vi "HFRR ADV v024 new software.vi"() -> ()   [LabVIEW 2025] (continued)
            n3097 = local write "OK Button 17"(FALSE ("OK Button 17")) -> ()
            n3098 = local read "String"() -> (w4300:string)
            n3099 = String To Path(string=w4300) -> (path=w4301:path)
            n3100 = File Dialog(6:"*.duf" ("pattern"), 7:w4305, 11:w4301) -> (0:w4292:errorcluster, 3:w4311:path)  [unwired: 4 in, 2 out]
            n3101 = Unbundle(w4292) -> ()  [unwired: 3 out]
            n3102 = Open/Create/Replace File "Open File"(file path (use dialog)=w4311) -> (refnum out=w4303:refnum<file>)  [unwired: 5 in, 2 out]
            n3103 = Strip Path(path=w4311) -> (name=w4309:string)  [unwired: 1 out]
            n3104 = Path To String(path=w4311) -> (string=w4294:string)
            n3105 = while {
              tunnel: w4303 -> [w4315]
              i -> [w4312]
              stop <- w4313 continue-if-true
              (unwired) TRUE ("line mode (F)")
              n3106 = Read from Text File "Read File"(file (use dialog)=w4315) -> (text=w4314:string)  [unwired: 3 in, 3 out]
              n3107 = local write "Numeric 16"(w4312) -> ()
              n3108 = String Length(string=w4314) -> (length=w4317:i32)
              n3109 = Greater?(x=w4317, y=1) -> (0:w4313:bool)
            }
            n3110 = local write "String 29"(w4294) -> ()
            n3111 = Search and Replace String(input string=w4294, search string=".duf", replace string=".dgf" ("replace string (\"\")")) -> (result string=→"String Indicator 4":string)  [unwired: 5 in, 3 out]
            n3112 = Match Pattern(string=w4309, regular expression=".dwm") -> (before substring=w4293:string)  [unwired: 1 in, 3 out]
            "String Indicator" <- w4293
            n3113 = Match Pattern(string=w4294, regular expression=".dwm" ("substring (\"\")")) -> (before substring=w4295:string)  [unwired: 1 in, 3 out]
            "String Indicator 3" <- w4295
            n3114 = local write "TITTLE 2"(w4293) -> ()
            n3115 = String To Path(string=w4295) -> (path=w4302:path)
            "path" <- w4302
            n3116 = call <vilib>:"Read Characters From File.vi"("file path (dialog if empty)"=w4302, "start of read offset (chars.:0)"=60 ("start of read offset (chars.: 0)")) -> ("character string"=→"String Indicator 2":string)  [unwired: 4 in, 3 out]
          }
        }
        n3117 = call <vilib>:"Query Available Printers.vi"() -> ("system configured printers"=w3994:string[])  [unwired: 9 in, 2 out]
        "System Configured Printers 2" <- w3994
        n3118 = local read "OK Button 16"() -> (w3991:bool)
        n3119 = case shown="True" "OK Button 16" {
          frame False {
          }
          frame True {
            n3120 = stacked-sequence {
              frame #0 {
                n3121 = local read "Numeric 16"() -> (w4319:i32)
                n3122 = local write "Numeric 10"(w4319) -> ()
              }
              frame #1 {
                n3123 = local read "S.NO"() -> (→"s.NO":string)
                n3124 = local read "String 29"() -> (w4323:string)
                n3125 = String To Path(string=w4323) -> (path=w4322:path)
                n3126 = Open/Create/Replace File "Open File"(file path (use dialog)=w4322) -> (refnum out=w4324:refnum<file>)  [unwired: 5 in, 2 out]
                n3127 = for {
                  N: 16 -> [_]
                  tunnel: w4324 -> [w4331]
                  i -> [w4327]
                  (unwired) TRUE ("line mode (F)")
                  n3128 = Read from Text File "Read File"(file (use dialog)=w4331) -> (text=w4325:string)  [unwired: 3 in, 3 out]
                  n3129 = Match Pattern(string=w4325, regular expression="(") -> (after substring=w4330:string)  [unwired: 1 in, 3 out]
                  n3130 = Match Pattern(string=w4330, regular expression=")") -> (before substring=w4326:string)  [unwired: 1 in, 3 out]
                  n3131 = case shown="1" w4327 {
                    tunnel: w4326 -> [w4332 w4333 _ _ w4334 w4335 w4336 w4338 w4340 w4342 w4344 w4346 w4348 w4350 _]
                    tunnel: w4325 -> [_ _ _ _ _ _ _ _ _ _ _ _ _ _ _]
                    frame 0 {
                      "TITTLE" <- w4332
                    }
                    frame 1 {
                      "Sample ID" <- w4333
                    }
                    frame 2 {
                    }
                    frame 3 {
                    }
                    frame 4 {
                      "Test Date" <- w4334
                    }
                    frame 5 {
                      "Tested by" <- w4335
                    }
                    frame 6 {
                      n3132 = Fract/Exp String To Number(string=w4336) -> (number=→"Humidity before test 2":dbl)  [unwired: 3 in, 1 out]
                    }
                    frame 7 {
                      n3133 = Fract/Exp String To Number(string=w4338) -> (number=→"Temperature before test 2":dbl)  [unwired: 3 in, 1 out]
                    }
                    frame 8 {
                      n3134 = Fract/Exp String To Number(string=w4340) -> (number=→"Humidity after test 2":dbl)  [unwired: 3 in, 1 out]
                    }
                    frame 9 {
                      n3135 = Fract/Exp String To Number(string=w4342) -> (number=→"Temperature after test 2":dbl)  [unwired: 3 in, 1 out]
                    }
                    frame 10 {
                      n3136 = Fract/Exp String To Number(string=w4344) -> (number=→"MWSD 2":dbl)  [unwired: 3 in, 1 out]
                    }
                    frame 11 {
                      n3137 = Fract/Exp String To Number(string=w4346) -> (number=→"AVP 2":dbl)  [unwired: 3 in, 1 out]
                    }
                    frame 12 {
                      n3138 = Fract/Exp String To Number(string=w4348) -> (number=→"HCF 2":dbl)  [unwired: 3 in, 1 out]
                    }
                    frame 13 {
                      n3139 = Fract/Exp String To Number(string=w4350) -> (number=→"WS1.4 2":dbl)  [unwired: 3 in, 1 out]
                    }
                    frame 14, Default {
                    }
                  }
                }
              }
              frame #2 {
              }
            }
            n3140 = local write "OK Button 16"(FALSE ("OK Button 13")) -> ()
          }
        }
        n3141 = Index Array(array=w3994, index="Select Printer 3") -> (element=w3996:string)
        "Selected Printer" <- w3996
        n3142 = case shown="True" w3991 {
          frame False {
          }
          frame True {
            n3143 = flat-sequence {
              frame #0 {
              }
              frame #1 {
                n3144 = Wait (ms)(milliseconds to wait=u32 100) -> ()  [unwired: 1 out]
              }
              frame #2 {
                n3145 = local write "OK Button 16"(FALSE ("Print 3")) -> ()
              }
            }
          }
        }
        n3146 = case shown="True" "Print" {
          tunnel: w3996 -> [_ w4288]
          frame False {
          }
          frame True {
            (unwired) i16 6 ("width (-)")
            (unwired) "TESTED BY : "
            (unwired) "TESTED DATE :"
            (unwired) "SAMPLE ID : "
            (unwired) "SAMPLE DESIGN : "
            w4246 = "\r"
            w4263 = "\r"
            # "add image"
            n3147 = local read "Sample ID"() -> (w4236:string)
            n3148 = local read "Tested by"() -> (w4239:string)
            n3149 = local read "String 34"() -> (w4226:string)
            n3150 = local read "String 45"() -> (w4206:string)
            n3151 = local read "String 35"() -> (w4221:string)
            n3152 = local read "String 37"() -> (w4219:string)
            n3153 = local read "String 32"() -> (w4241:string)
            n3154 = local read "String 36"() -> (w4216:string)
            n3155 = local read "String 31"() -> (w4240:string)
            n3156 = local read "Test Date"() -> (w4237:string)
            n3157 = local read "String 33"() -> (w4242:string)
            n3158 = local read "String 38"() -> (w4212:string)
            n3159 = local read "String 39"() -> (w4209:string)
            n3160 = local write "Print"(FALSE ("Print FF")) -> ()
            n3161 = local read "S 39"() -> (w4224:string)
            n3162 = local read "S 38"() -> (w4231:string)
            n3163 = local read "Temperature before test 2"() -> (w4262:dbl)
            n3164 = local read "Temperature after test 2"() -> (w4252:dbl)
            n3165 = local read "Humidity before test 2"() -> (w4277:dbl)
            n3166 = local read "Humidity after test 2"() -> (w4261:dbl)
            n3167 = local read "MWSD 2"() -> (w4266:dbl)
            n3168 = local read "WS1.4 2"() -> (w4244:dbl)
            n3169 = Concatenate Strings("2)" ("string"), w4226) -> (w4227:string)
            n3170 = Concatenate Strings("3)" ("string"), w4224) -> (w4225:string)
            n3171 = Concatenate Strings("1)" ("string"), w4231) -> (w4230:string)
            n3172 = Concatenate Strings("4)" ("string"), w4221) -> (w4222:string)
            n3173 = Concatenate Strings("5)" ("string"), w4219) -> (w4218:string)
            n3174 = Concatenate Strings("6)" ("string"), w4216) -> (w4215:string)
            n3175 = Concatenate Strings("7)" ("string"), w4212) -> (w4213:string)
            n3176 = Concatenate Strings("8)" ("string"), w4209) -> (w4210:string)
            n3177 = local read "HCF 2"() -> (w4248:dbl)
            n3178 = local read "AVP 2"() -> (w4265:dbl)
            n3179 = local read "s.NO"() -> (w4207:string)
            n3180 = call <vilib>:"New Report.vi"("report type"=enum16{"Standard Report", "HTML"}."Standard Report") -> ("report out"=w4286:refnum<class "NI_report.lvclass">, "error out"=w4285:errorcluster)  [unwired: 13 in]
            n3181 = local read "TITTLE"() -> (w4238:string)
            n3182 = Concatenate Strings(w4263, w4206, w4207, w4263, w4241, w4236, w4263, w4240, w4237, w4263, w4242, w4239, w4263) -> (w4256:string)
            "test by" <- w4256
            n3183 = Number To Fractional String(number=w4262, width (-)=i16 6, precision (6)=i16 2) -> (F-format string=w4251:string)  [unwired: 1 in]
            n3184 = Number To Fractional String(number=w4261, width (-)=i16 6, precision (6)=i16 2) -> (F-format string=w4264:string)  [unwired: 1 in]
            n3185 = Number To Fractional String(number=w4277, width (-)=i16 6, precision (6)=i16 2) -> (F-format string=w4282:string)  [unwired: 1 in]
            n3186 = Number To Fractional String(number=w4266, width (-)=i16 6, precision (6)=i16 2) -> (F-format string=w4268:string)  [unwired: 1 in]
            n3187 = Number To Fractional String(number=w4252, width (-)=i16 6, precision (6)=i16 2) -> (F-format string=w4253:string)  [unwired: 1 in]
            n3188 = Number To Fractional String(number=w4265, width (-)=i16 6, precision (6)=i16 2) -> (F-format string=w4267:string)  [unwired: 1 in]
            n3189 = Number To Fractional String(number=w4248, width (-)=i16 6, precision (6)=i16 2) -> (F-format string=w4247:string)  [unwired: 1 in]
            n3190 = Number To Fractional String(number=w4244, precision (6)=i16 2) -> (F-format string=w4243:string)  [unwired: 2 in]
            n3191 = call-dynamic "Set Report Header Text.vi"("report in"=w4286, "center header text"=w4238, "error in (no error)"=w4285) -> ("report out"=w4257:refnum<class "NI_report.lvclass">, "error out"=w4258:errorcluster)  [unwired: 11 in]
            n3192 = Concatenate Strings(w4246, w4230, w4282, w4246, w4227, w4251, w4246, w4225, w4264, w4246, w4222, w4253, w4246, w4218, w4268, w4246, w4215, w4267, w4246, w4213, w4247, w4246, w4210, w4243) -> (w4234:string)
            "export 2" <- w4234
            n3193 = call-poly <vilib>:"Append Report Text.vi"("report in"=w4257, "text"=w4256, "error in (no error)"=w4258) -> ("report out"=w4260:refnum<class "NI_report.lvclass">, "error out"=w4259:errorcluster)  [unwired: 9 in, 2 out]
            n3194 = local read "test by"() -> (w4233:string)
            n3195 = local read "TITTLE"() -> (w4235:string)
            n3196 = call-poly <vilib>:"Append Report Text.vi"("report in"=w4260, "error in (no error)"=w4259) -> ("report out"=w4281:refnum<class "NI_report.lvclass">, "error out"=w4279:errorcluster)  [unwired: 10 in, 2 out]
            n3197 = Concatenate Strings(w4235, w4234, w4233) -> (→"output":string)
            n3198 = call-poly <vilib>:"Append Report Text.vi"("report in"=w4281, "text"=w4234, "error in (no error)"=w4279) -> ("report out"=w4280:refnum<class "NI_report.lvclass">, "error out"=w4278:errorcluster)  [unwired: 9 in, 2 out]
            n3199 = call-dynamic "Print Report.vi"("report in"=w4280, "printer name (default)"=w4288, "error in (no error)"=w4278) -> ("report out"=w4290:refnum<class "NI_report.lvclass">, "error out"=w4291:errorcluster)  [unwired: 11 in]
            n3200 = call-dynamic "Dispose Report.vi"("report in"=w4290, "error in (no error)"=w4291) -> ()  [unwired: 13 in, 1 out]
          }
        }
        n3201 = case shown="True" "Print 2" {
          frame False {
          }
          frame True {
            n3202 = flat-sequence {
              frame #0 {
                n3203 = local read "s.NO"() -> (→"s.NO 2":string)
                n3204 = Wait (ms)(milliseconds to wait=u32 20) -> ()  [unwired: 1 out]
                n3205 = local read "Sample ID  3"() -> (→"Sample ID  6":string)
                n3206 = local read "Sample ID  4"() -> (→"Sample ID  7":string)
                n3207 = local read "Sample ID"() -> (→"Sample ID  2":string)
                n3208 = local read "Tested by"() -> (→"Tested by 2":string)
                n3209 = local read "Test Date"() -> (→"Test Date 2":string)
                n3210 = local read "Humidity after test 3"() -> (→"Humidity after test 4":dbl)
                n3211 = local read "Ref A Test Date :"() -> (→"TITTLE 4":string)
                n3212 = local read "Temperature before test 3"() -> (w4113:dbl)
                n3213 = local read "Temperature before test 3"() -> (→"Temperature after test 5":dbl)
                n3214 = local read "Temperature after test 3"() -> (→"Temperature after test 4":dbl)
                n3215 = local read "Humidity before test 3"() -> (→"Humidity before test 4":dbl)
                n3216 = local write "Temperature before test 3"(w4113) -> ()
                n3217 = local read "image data"() -> (w4104:T16)
                n3218 = String To Path(string="C:\\LAB-IQ\\im\\Temp_resized.jpg") -> (path=w4105:path)
                "path 2" <- w4105
                n3219 = call <vilib>:"Write JPEG File.vi"("image data"=w4104, "path to JPEG file"=w4105) -> ()  [unwired: 8 in, 2 out]
                "Ref A Test Date :" <- "Ref A Test Date :"
                "Ref B Test Date :" <- "Ref B Test Date :"
                "Ref B Scar Value :" <- "Ref B Scar Value :"
                "Ref A Scar Value :" <- "Ref A Scar Value :"
              }
              frame #1 {
                (unwired) HTML_Report_Image_Alignment."MIDDLE" ("alignment (default)")
                w4141 = u16 0 items=["portrait", "landscape"] ("orientation (portrait)")
                (unwired) HTML_Report_Image_Alignment."ABSMIDDLE" ("alignment (default)")
                (unwired) "TESTED BY : "
                (unwired) "TESTED DATE :"
                (unwired) "SAMPLE ID : "
                (unwired) "SAMPLE DESIGN : "
                w4174 = "\r"
                # "add image"
                n3220 = Wait (ms)(milliseconds to wait=u32 20) -> ()  [unwired: 1 out]
                n3221 = local read "Sample ID  2"() -> (w4167:string)
                n3222 = local read "Wear Scar X"() -> (w4139:dbl)
                "Length ( microns ) 2" <- w4139
                n3223 = local read "Wear Scar Y"() -> (w4138:dbl)
                "Wear Scar Y ( microns ) :" <- w4138
                n3224 = local read "Test Date 2"() -> (w4168:string)
                n3225 = local read "Tested by 2"() -> (w4169:string)
                n3226 = local read "String 46"() -> (w4165:string)
                n3227 = local read "String 48"() -> (w4171:string)
                n3228 = local read "String 47"() -> (w4170:string)
                n3229 = local read "String 49"() -> (w4172:string)
                n3230 = local read "String 10"() -> (w4125:string)
                n3231 = local read "s.NO 2"() -> (w4166:string)
                n3232 = Add(x=w4139, y=w4138) -> (x+y=w4137:dbl)
                n3233 = call <vilib>:"New Report.vi"("report type"=enum16{"Standard Report", "HTML"}."HTML") -> ("report out"=w4145:refnum<class "NI_report.lvclass">, "error out"=w4143:errorcluster)  [unwired: 13 in]
                n3234 = Concatenate Strings(w4174, w4165, w4166, w4174, w4171, w4167, w4174, w4170, w4168, w4174, w4172, w4169, w4174) -> (→"test by 2":string)
                n3235 = Concatenate Strings("C:\\LAB-IQ\\Data\\" ("string"), w4125, ".jpg" ("string")) -> ()  [unwired: 1 out]
                n3236 = Divide(x=w4137, y=2.0) -> (x/y=→"Mean Wear ( microns) :":dbl)
                n3237 = call-dynamic "Set Report Orientation.vi"("report in"=w4145, "orientation (portrait)"=w4141, "error in (no error)"=w4143) -> ("report out"=w4144:refnum<class "NI_report.lvclass">, "error out"=w4142:errorcluster)  [unwired: 11 in]
                n3238 = for {
                  N: 5 -> [_]
                  tunnel: w4144 -> [w4195]
                  tunnel: [w4194] -> w4123
                  tunnel: w4142 -> [w4193]
                  tunnel: [w4192] -> w4122
                  n3239 = call-dynamic "Set Report Tab Width.vi"("report in"=w4195, "error in (no error)"=w4193) -> ("report out"=w4194:refnum<class "NI_report.lvclass">, "error out"=w4192:errorcluster)  [unwired: 12 in]
                }
                n3240 = local read "TITTLE"() -> (w4140:string)
                n3241 = call-dynamic "Set Report Header Text.vi"("report in"=w4123, "center header text"=w4140, "error in (no error)"=w4122) -> ("report out"=w4161:refnum<class "NI_report.lvclass">, "error out"=w4160:errorcluster)  [unwired: 11 in]
                n3242 = for {
                  N: 1 -> [_]
                  tunnel: [w4199] -> w4147
                  tunnel: [w4198] -> w4146
                  tunnel: w4161 -> [w4197]
                  tunnel: w4160 -> [w4196]
                  n3243 = call-dynamic "New Report Line.vi"("report in"=w4197, "error in (no error)"=w4196) -> ("report out"=w4199:refnum<class "NI_report.lvclass">, "error out"=w4198:errorcluster)  [unwired: 12 in]
                }
                n3244 = for {
                  N: 2 -> [_]
                  tunnel: [w4191] -> w4153
                  tunnel: [w4190] -> w4152
                  tunnel: w4147 -> [w4189]
                  tunnel: w4146 -> [w4188]
                  n3245 = call-dynamic "New Report Line.vi"("report in"=w4189, "error in (no error)"=w4188) -> ("report out"=w4191:refnum<class "NI_report.lvclass">, "error out"=w4190:errorcluster)  [unwired: 12 in]
                }
                n3246 = for {
                  N: 25 -> [_]
                  tunnel: w4153 -> [w4187]
                  tunnel: w4152 -> [w4185]
                  tunnel: [w4186] -> w4156
                  tunnel: [w4184] -> w4155
                  n3247 = call-dynamic "Set Report Tab Width.vi"("report in"=w4187, "error in (no error)"=w4185) -> ("report out"=w4186:refnum<class "NI_report.lvclass">, "error out"=w4184:errorcluster)  [unwired: 12 in]
                }
                n3248 = control-ref of="Tab Control 9"() -> (w4151:refnum<vi>)
                n3249 = call-dynamic "Append Control Image to Report.vi"("report in"=w4156, "alignment (default)"=HTML_Report_Image_Alignment."ABSMIDDLE", "ctrl reference"=w4151, "error in (no error)"=w4155) -> ("report out"=w4150:refnum<class "NI_report.lvclass">, "error out"=w4149:errorcluster)  [unwired: 8 in, 2 out]
                n3250 = for {
                  N: 3 -> [_]
                  tunnel: [w4183] -> w4134
                  tunnel: [w4182] -> w4133
                  tunnel: w4150 -> [w4181]
                  tunnel: w4149 -> [w4180]
                  n3251 = call-dynamic "New Report Line.vi"("report in"=w4181, "error in (no error)"=w4180) -> ("report out"=w4183:refnum<class "NI_report.lvclass">, "error out"=w4182:errorcluster)  [unwired: 12 in]
                }
                n3252 = for {
                  N: 100 -> [_]
                  tunnel: w4134 -> [w4179]
                  tunnel: w4133 -> [w4177]
                  tunnel: [w4178] -> w4130
                  tunnel: [w4176] -> w4128
                  n3253 = call-dynamic "Set Report Tab Width.vi"("report in"=w4179, "error in (no error)"=w4177) -> ("report out"=w4178:refnum<class "NI_report.lvclass">, "error out"=w4176:errorcluster)  [unwired: 12 in]
                }
                n3254 = String To Path(string="C:\\LAB-IQ\\im\\Temp_resized.jpg") -> (path=w4120:path)
                n3255 = call-poly <vilib>:"Append Image to Report.vi"("report in"=w4130, "path or URL of image"=w4120, "error in (no error)"=w4128) -> ("report out"=w4129:refnum<class "NI_report.lvclass">, "error out"=w4127:errorcluster)  [unwired: 9 in, 2 out]
                n3256 = call-poly <vilib>:"Open HTML Report in Browser.vi"("report in"=w4129, "error in (no error)"=w4127) -> ("report out"=w4164:refnum<class "NI_report.lvclass">, "error out"=w4163:errorcluster)  [unwired: 11 in, 1 out]
                n3257 = call-dynamic "Dispose Report.vi"("report in"=w4164, "error in (no error)"=w4163) -> ()  [unwired: 13 in, 1 out]
              }
              frame #2 {
              }
              frame #3 {
                n3258 = disable-structure shown="Disabled" {
                  frame Disabled {
                    n3259 = local read "String 10"() -> (w4204:string)
                    n3260 = Concatenate Strings("C:\\LAB-IQ-NXT\\Data\\" ("string"), w4204, ".jpg" ("string")) -> (w4202:string)
                    n3261 = String To Path(string=w4202) -> (path=w4201:path)
                    n3262 = Delete(path (use dialog)=w4201) -> ()  [unwired: 4 in, 3 out]
                  }
                  frame Enabled {
                  }
                }
                n3263 = local write "Print 2"(FALSE ("Print")) -> ()
              }
            }
          }
        }
      }
    }
    n3264 = property on="SetTemp" class="DigNum (strict)"("Disabled"=w2147) -> ()  [unwired: 2 in, 2 out]
    n3265 = Multiply(x=w2137, y=w2139) -> (x*y=w2138:dbl)
    n3266 = local read "MWSD"() -> (w2136:dbl)
    n3267 = Add(x=w2138, y=w2136) -> (x+y=→"WS1.4":dbl)
    n3268 = Wait (ms)(milliseconds to wait=u32 50) -> ()  [unwired: 1 out]
    n3269 = Wait (ms)(milliseconds to wait=u32 50) -> ()  [unwired: 1 out]
    n3270 = local read "Quit"() -> (w2135:bool)
  }
  n3271 = VISA Close(VISA resource name=w44, error in (no error)=w43) -> ()  [unwired: 1 out]
  n3272 = while {
    tunnel: [w4365] -> w53
    shift-right: [w4358] -> _
    shift-left: 0.0 -> [w4361]
    shift-right: [w4357] -> _
    shift-left: 0.0 -> [w4360]
    shift-right: [w4356] -> _
    shift-left: 100.0 ("vc_cmd") -> [w4359]
    stop <- w4365 stop-if-true
    # "PID LOGIC"
    n3273 = local read "RUN"() -> (w4363:bool)
    n3274 = local read "Auto Start Temp"() -> (w4352:bool)
    n3275 = local read "Auto Start Test"() -> (w4362:bool)
    n3276 = local read "START TEMP"() -> (w4354:bool)
    n3277 = And(x=w4352, y=w4362) -> (x .and. y?=w4353:bool)
    n3278 = Or(x=w4363, y=w4353) -> (x .or. y?=w4364:bool)
    n3279 = And(x=w4364, y=w4354) -> (x .and. y?=w4355:bool)
    n3280 = Wait (ms)(milliseconds to wait="milliseconds to wait") -> ()  [unwired: 1 out]
    n3281 = case shown="True" w4355 {
      tunnel: [400.0 ("out_vc_cmd") w4385] -> w4356
      tunnel: [w4368 w4387] -> w4357
      tunnel: [w4368 w4386] -> w4358
      tunnel: w4361 -> [_ w4376]
      tunnel: w4360 -> [_ w4375]
      tunnel: w4359 -> [_ w4374]
      frame False {
        w4368 = 0.0 ("error_out")
      }
      frame True {
        n3282 = local read "Set Strk"() -> (w4371:dbl)
        n3283 = local read "LVDT STROKE"() -> (w4369:dbl)
        n3284 = Add(x=w4371, y="Add up Stroke") -> (x+y=w4372:dbl)
        n3285 = formula code="// Zero-Hardcode Explicit Positional-Form PID Engine\n// Inputs: target_stroke, measured_stroke, dt, prev_error, integral_accumulator_in, prev_vc_cmd\n//         kp, ki, kd, max_step_change, max_amplitude, min_amplitude, startup_cmd\n// Outputs: vc_cmd, error_out, out_error, integral_accumulator_out, out_vc_cmd\n\n// 1. Calculate Tracking Error\nfloat current_error = target_stroke - measured_stroke;\nerror_out = current_error;\n\n// 2. Compute Proportional Term\nfloat p_term = kp * current_error;\n\n// 3. Compute Derivative Term\nfloat d_term = 0.0;\nif (dt > 0.0) {\n    d_term = kd * ((current_error - prev_error) / dt);\n}\n\n// 4. Update and Accumulate Integral Term\nfloat current_integral = integral_accumulator_in + (current_error * dt);\nfloat i_term = ki * current_integral;\n\n// 5. Calculate Ideal Target Command\nfloat ideal_command = startup_cmd + p_term + i_term + d_term;\n\n// 6. Anti-Windup Protection (Back-calculation method)\nif (ideal_command > max_amplitude) {\n    float excess = ideal_command - max_amplitude;\n    if (ki > 0.0) {\n        current_integral -= excess / ki;\n    }\n    ideal_command = max_amplitude;\n} else if (ideal_command < min_amplitude) {\n    float excess = ideal_command - min_amplitude;\n    if (ki > 0.0) {\n        current_integral -= excess / ki;\n    }\n    ideal_command = min_amplitude;\n}\n\n// 7. Apply Loop Rate Limiting (Protects voice coil from large voltage steps)\nfloat raw_adjustment = ideal_command - prev_vc_cmd;\n\nif (raw_adjustment > max_step_change) {\n    raw_adjustment = max_step_change;\n} else if (raw_adjustment < -max_step_change) {\n    raw_adjustment = -max_step_change;\n}\n\nfloat next_vc_cmd = prev_vc_cmd + raw_adjustment;\n\n// Final Output Safety Safeguard Clamping\nif (next_vc_cmd > max_amplitude) {\n    next_vc_cmd = max_amplitude;\n} else if (next_vc_cmd < min_amplitude) {\n    next_vc_cmd = min_amplitude;\n}\n\n// 8. Map to Shift Registers for memory persistence\nvc_cmd = next_vc_cmd;\nout_error = current_error;                     \nintegral_accumulator_out = current_integral;  \nout_vc_cmd = next_vc_cmd;"("target_stroke"=w4372, "measured_stroke"=w4369, "dt"="dt", "integral_accumulator_in"=w4375, "prev_error"=w4376, "prev_vc_cmd"=w4374, "kp"="kp", "ki"="ki", "kd"="kd", "max_step_change"="max_step_change", "max_amplitude"="max_amplitude", "min_amplitude"="min_amplitude", "startup_cmd"="startup_cmd") -> ("vc_cmd"=w4391:dbl, "out_error"=w4386:dbl, "integral_accumulator_out"=w4387:dbl, "out_vc_cmd"=w4385:dbl)  [unwired: 1 out]
        "output Vpp" <- w4391
        n3286 = Number To Fractional String(number=w4391, precision (6)=i16 1) -> (F-format string=w4389:string)  [unwired: 2 in]
        n3287 = Concatenate Strings("DAC;" ("string"), w4389) -> (w4373:string)
        n3288 = local write "Due Write"(w4373) -> ()
        "prev_error" <- w4376
        "integral_accumulator_in" <- w4375
        "prev_vc_cmd" <- w4374
      }
    }
    n3289 = local read "Quit"() -> (w4365:bool)
  }
  n3290 = Or(x=w49, y=w48) -> (x .or. y?=w50:bool)
  n3291 = Or(x=w46, y=w50) -> (x .or. y?=w55:bool)
  n3292 = control-ref of="new picture"() -> ()  [unwired: 1 out]
  n3293 = Or(x=w58, y=w55) -> (x .or. y?=w52:bool)
  n3294 = Or(x=w52, y=w53) -> (x .or. y?=w47:bool)
  n3295 = while {
    tunnel: [w4392] -> w57
    i -> [w4399]
    stop <- w4392 stop-if-true
    n3296 = local read "Quit"() -> (w4392:bool)
    n3297 = Equal To 0?(x=w4399) -> (x = 0?=w4397:bool)
    n3298 = call "Elapsed Time3"("Time Target (s)"=45.0, "Auto Reset"=TRUE) -> ("Time has Elapsed"=w4396:bool)  [unwired: 10 in, 7 out]
    n3299 = Wait (ms)(milliseconds to wait=u32 50) -> ()  [unwired: 1 out]
    n3300 = Or(x=w4396, y=w4397) -> (x .or. y?=w4398:bool)
    n3301 = case shown="True" w4398 {
      frame False {
      }
      frame True {
        n3302 = call <vilib>:"System Exec.vi"("run minimized? (F)"=TRUE, "error in (no error)"="error in (no error)", "command line"="powercfg.exe -change -monitor-timeout-ac 0") -> ("error out"=w4410:errorcluster)  [unwired: 5 in, 3 out]
        n3303 = call <vilib>:"System Exec.vi"("run minimized? (F)"=TRUE, "error in (no error)"=w4410, "command line"="powercfg.exe -change -disk-timeout-ac 0") -> ("error out"=w4409:errorcluster)  [unwired: 5 in, 3 out]
        n3304 = call <vilib>:"System Exec.vi"("run minimized? (F)"=TRUE, "error in (no error)"=w4409, "command line"="powercfg.exe -change -standby-timeout-ac 0") -> ("error out"=w4408:errorcluster)  [unwired: 5 in, 3 out]
        n3305 = call <vilib>:"System Exec.vi"("run minimized? (F)"=TRUE, "error in (no error)"=w4408, "command line"="powercfg.exe -change -hibernate-timeout-ac 0") -> ("error out"=w4407:errorcluster)  [unwired: 5 in, 3 out]
        n3306 = call <vilib>:"Simple Error Handler.vi"("error in (no error)"=w4407) -> ("error out"=w4413:errorcluster)  [unwired: 4 in, 4 out]
        n3307 = call <vilib>:"Clear Errors.vi"("error in (no error)"=w4413) -> ("error out"=→"error out":errorcluster)  [unwired: 5 in, 1 out]
      }
    }
  }
  n3308 = Compound Arithmetic op=OR(w60, w47, w57) -> (w59:bool)
  n3309 = flat-sequence {
    tunnel: w59 -> [_]
    tunnel: [w4415] -> w25
    tunnel: w25 -> [_]
    frame #0 {
      n3310 = call "CLOSE CONNECTION.vi"() -> ("error out"=w4415:errorcluster)  [unwired: 11 in]
    }
    frame #1 {
      n3311 = Quit LabVIEW(quit? (T)=TRUE) -> ()
      n3312 = local write "Quit"(FALSE ("EXIT")) -> ()
    }
  }
  n3313 = property on="Heater Button" class="Bool (strict)"("Visible"=TRUE) -> ()  [unwired: 2 in, 2 out]
  n3314 = disable-structure shown="Disabled" {
    disable-tunnel: _ -> [w4421 _]
    disable-tunnel: _ -> [w4418 _]
    disable-tunnel: _ -> [w4419 _]
    frame Disabled {
      n3315 = disable-structure shown="Disabled" {
        disable-tunnel: [w4428 _] -> w4420
        frame Disabled {
          n3316 = while {
            shift-right: [w4470] -> w4426
            shift-left: errorcluster {"status"=TRUE, "code"=0, "source"="Init"} ("error out") -> [w4435]
            shift-right: [w4469] -> w4425
            shift-left: _ -> [w4436]
            shift-right: [w4468] -> _
            shift-left: "" -> [w4467]
            tunnel: [w4429] -> w4428
            shift-right: ["Set Rh"] -> _
            shift-left: 0.0 ("Set Rh") -> [w4461]
            tunnel: [w4438] -> _
            i -> [w4438]
            stop <- w4429 stop-if-true
            n3317 = flat-sequence {
              tunnel: w4435 -> [w4473]
              tunnel: [w4473] -> w4434
              frame #0 {
                n3318 = Wait (ms)(milliseconds to wait=u32 200) -> ()  [unwired: 1 out]
              }
            }
            n3319 = local read "Com Port 3"() -> (w4437:refnum<visa-resource-name>)
            n3320 = local read "Humidity Str Rec"() -> (w4439:string)
            n3321 = Not Equal?(x="Set Rh", y=w4461) -> (x != y?=w4466:bool)
            n3322 = Number To Decimal String(number="Set Rh") -> (decimal integer string=w4464:string)  [unwired: 1 in]
            n3323 = Not Equal?(x=w4437, y=w4436) -> (x != y?=w4432:bool)
            n3324 = Concatenate Strings("#setPoint00" ("string"), w4464) -> (w4465:string)
            n3325 = case shown="False" w4466 {
              tunnel: w4465 -> [_ w4485]
              frame False {
                n3326 = local read "Humidity"() -> (w4482:bool)
                n3327 = case shown="True" w4482 {
                  frame False {
                    n3328 = local write "Humidity Str Send"("stop" ("Humidity Str Send")) -> ()
                  }
                  frame True {
                    n3329 = local write "Humidity Str Send"("start" ("Humidity Str Send")) -> ()
                  }
                }
              }
              frame True {
                n3330 = local write "Humidity Str Send"(w4485) -> ()
              }
            }
            n3331 = Or(x=w4432) -> (y=w4430:bool, x .or. y?=w4431:bool)
            n3332 = String Subset(string=w4439, offset (0)=7) -> (substring=w4454:string)  [unwired: 1 in]
            n3333 = Match Pattern(string=w4439, regular expression="?") -> (offset past match=w4457:i32)  [unwired: 1 in, 3 out]
            n3334 = Match Pattern(string=w4439, regular expression="v") -> (offset past match=w4460:i32)  [unwired: 1 in, 3 out]
            n3335 = case shown="True" w4431 {
              tunnel: w4434 -> [w4471 _]
              tunnel: [w4471 errorcluster {"status"=TRUE, "code"=0, "source"="Init"} ("error out")] -> w4433
              frame False {
              }
              frame True {
              }
            }
            n3336 = Equal?(x=w4457, y=-1) -> (x = y?=w4441:bool)
            n3337 = Match Pattern(string=w4454, regular expression="g") -> (after substring=w4455:string, offset past match=w4446:i32)  [unwired: 1 in, 2 out]
            n3338 = Match Pattern(string=w4454, regular expression="y") -> (after substring=w4453:string, offset past match=w4447:i32)  [unwired: 1 in, 2 out]
            n3339 = Greater?(x=w4447, y=w4446) -> (0:w4452:bool)
            n3340 = Greater Or Equal To 0?(x=w4447) -> (x >= 0?=w4444:bool)
            n3341 = Greater Or Equal To 0?(x=w4446) -> (x >= 0?=w4445:bool)
            n3342 = Or(x=w4444, y=w4445) -> (x .or. y?=w4443:bool)
            n3343 = Greater Or Equal To 0?(x=w4460) -> (x >= 0?=w4442:bool)
            n3344 = Select(t=w4453, s=w4452, f=w4455) -> (s? t:f=w4448:string)
            n3345 = case shown="Error" w4433 {
              selector: w4433 -> [w4498 w4544]
              tunnel: [w4496 w4537] -> w4470
              tunnel: w4436 -> [w4499 w4543]
              tunnel: [w4497 w4546] -> w4469
              tunnel: w4467 -> [w4486 w4545]
              tunnel: [w4493 w4545] -> w4468
              frame No Error {
                n3346 = call "Elapsed Time7"() -> ("Time has Elapsed"=w4492:bool)  [unwired: 12 in, 7 out]
                n3347 = Not Equal?(x="Humidity Str Send", y=w4486) -> (x != y?=w4488:bool)
                n3348 = Or(x=w4488, y=w4492) -> (x .or. y?=w4491:bool)
                n3349 = Select(t="Humidity Str Send", s=w4488, f="vals" ("regular expression")) -> (s? t:f=w4487:string)
                n3350 = Or(x=w4491, y="Send") -> (x .or. y?=w4495:bool)
                n3351 = case shown="True" w4495 {
                  tunnel: [w4502 w4507] -> w4496
                  tunnel: w4499 -> [w4501 w4515]
                  tunnel: w4498 -> [w4502 w4514]
                  tunnel: [w4501 w4508] -> w4497
                  tunnel: w4487 -> [_ w4513]
                  tunnel: [w4500 w4504] -> w4493
                  tunnel: "Humidity Str Send" -> [_ w4505]
                  tunnel: w4488 -> [_ w4506]
                  tunnel: w4486 -> [w4500 w4503]
                  frame False {
                  }
                  frame True {
                    n3352 = flat-sequence {
                      tunnel: w4515 -> [w4523]
                      tunnel: w4514 -> [w4522]
                      tunnel: w4513 -> [w4519]
                      tunnel: [w4521] -> w4512
                      tunnel: [w4520] -> w4511
                      tunnel: w4512 -> [w4526]
                      tunnel: w4511 -> [w4525]
                      tunnel: [w4526] -> w4510
                      tunnel: [w4525] -> w4509
                      tunnel: w4510 -> [w4533]
                      tunnel: w4509 -> [w4532]
                      tunnel: [w4531] -> w4508
                      tunnel: [w4530] -> w4507
                      frame #0 {
                        n3353 = local write "Ser Led"(TRUE ("Boolean 4")) -> ()
                        n3354 = Concatenate Strings(w4519, "\r") -> (w4518:string)
                        n3355 = VISA Write(VISA resource name=w4523, write buffer=w4518, error in (no error)=w4522) -> (VISA resource name out=w4521:refnum<visa-resource-name>, error out=w4520:errorcluster)  [unwired: 1 out]
                      }
                      frame #1 {
                        n3356 = Wait (ms)(milliseconds to wait="wait") -> ()  [unwired: 1 out]
                      }
                      frame #2 {
                        w4528 = FALSE ("Send")
                        n3357 = property class="Instr"(reference=w4533, error in=w4532) -> (reference out=w4534:refnum<visa-resource-name>, error out=w4535:errorcluster, "Serial Settings:Number of Bytes at Serial Port"=w4527:u32)
                        n3358 = local write "Send"(w4528) -> ()
                        n3359 = local write "Ser Led"(w4528) -> ()
                        n3360 = VISA Read(VISA resource name=w4534, byte count=w4527, error in (no error)=w4535) -> (VISA resource name out=w4531:refnum<visa-resource-name>, read buffer=→"Humidity Str Rec":string, error out=w4530:errorcluster)  [unwired: 1 out]
                      }
                    }
                    n3361 = Select(t=w4505, s=w4506, f=w4503) -> (s? t:f=w4504:string)
                  }
                }
              }
              frame Error {
                w4551 = u16 0 items=["None"=0, "XON/XOFF"=1, "RTS/CTS"=2, "DTR/DSR"=4] ("flow control")
                w4547 = u16 0 items=["None", "Odd", "Even", "Mark", "Space"] ("parity")
                w4550 = u16 10 items=["1.0"=10, "1.5"=15, "2.0"=20] ("stop bits")
                n3362 = VISA Close(VISA resource name=w4543, error in (no error)=w4544) -> (error out=w4542:errorcluster)
                n3363 = local write "humid"("" ("humid")) -> ()
                n3364 = local write "Humidity Str Rec"("" ("Humidity Str Rec")) -> ()
                n3365 = call <vilib>:"Clear Errors.vi"("error in (no error)"=w4542) -> ("error out"=w4541:errorcluster)  [unwired: 5 in, 1 out]
                n3366 = local read "Com Port 3"() -> (w4540:refnum<visa-resource-name>)
                n3367 = call-poly "VISA Configure Serial Port"("VISA resource name"=w4540, "timeout (10sec)"=u32 1000, "termination char\n(0xA = '\\n' = LF)"=u8 10 ("termination char\n(0xA = '\\n' = LF)"), "Enable Termination\nChar (T)"=FALSE ("Enable Termination Char (T)"), "data bits (8)"=u16 8 ("data bits"), "parity (0:none)"=w4547, "error in (no error)"=w4541, "stop bits (10: 1 bit)"=w4550, "flow control (0:none)"=w4551) -> ("VISA resource name out"=w4546:refnum<visa-resource-name>, "baud rate (9600)"=w4538:u32, "error out"=w4537:errorcluster)  [unwired: 4 in]
              }
            }
            n3368 = Compound Arithmetic op=AND(w4442, w4441, w4443) -> (w4440:bool)
            n3369 = case shown="True" w4440 {
              tunnel: w4439 -> [_ _]
              tunnel: w4448 -> [_ w4478]
              frame False {
              }
              frame True {
                w4476 = " " ("regular expression")
                n3370 = Match Pattern(string=w4478, regular expression=" ") -> (after substring=w4480:string)  [unwired: 1 in, 3 out]
                n3371 = Match Pattern(string=w4480, regular expression=w4476) -> (before substring=→"humid":string, after substring=w4477:string)  [unwired: 1 in, 2 out]
                n3372 = Match Pattern(string=w4477, regular expression=w4476) -> (before substring=→"temp_@Rh sensor":string)  [unwired: 1 in, 3 out]
              }
            }
            n3373 = local read "Quit"() -> (w4429:bool)
          }
          n3374 = VISA Close(VISA resource name=w4425, error in (no error)=w4426) -> (error out=w4422:errorcluster)
          n3375 = call <vilib>:"Clear Errors.vi"("error in (no error)"=w4422) -> ()  [unwired: 5 in, 2 out]
        }
        frame Enabled {
        }
      }
    }
    frame Enabled {
    }
  }
  n3376 = while {
    tunnel: [w4558] -> _
    i -> [w4558]
    stop <- w4554 stop-if-true
    # "Langauage selection"
    n3377 = Equal?(x="Lan flag", y=22.0) -> ()  [unwired: 1 out]
    n3378 = disable-structure shown="Disabled" {
      frame Disabled {
        n3379 = stacked-sequence {
          frame #0 {
            n3380 = case shown="\"Russian\"" "Language Selection" {
              tunnel: [0 1] -> w4560
              frame "English", Default {
              }
              frame "Russian" {
              }
            }
            n3381 = for {
              N: 130 -> [_]
              tunnel: "Table" -> [w4569]
              tunnel: w4560 -> [w4568]
              i -> [w4567]
              n3382 = Index Array(array=w4569, index (row)=w4567, index (col)=w4568) -> (element=w4566:string)
              n3383 = case shown="123" w4567 {
                tunnel: w4566 -> [w4570 w4571 _ w4572 w4573 w4574 w4575 w4576 w4577 w4578 w4579 w4580 w4581 w4582 w4583 w4584 w4585 w4586 w4587 w4588 w4589 w4590 w4591 w4592 w4593 w4594 w4595 w4596 w4597 _ _ w4598 w4599 w4600 w4601 w4602 w4603 w4612 w4619 w4626 w4633 w4637 w4640 w4643 w4645 w4647 w4648 w4649 w4650 w4651 w4652 w4653 w4654 w4655 w4656 w4657 w4658 w4659 w4660 w4661 w4662 w4663 w4664 w4665 w4666 w4667 w4668 w4669 w4670 w4671 w4672 w4673 w4674 w4675 w4676 w4677 w4678 w4679 w4680 w4681 w4682 w4683 w4684 w4685 w4686 w4687 w4688 w4689 w4690 w4691 w4692 w4693 w4694 w4695 w4696 w4697 w4698 w4699 w4700 w4701 w4702 w4703 w4704 w4705 w4706 _ w4707 w4708 w4709 w4710 w4711 w4712 w4713 w4714 w4715 w4716 w4717 w4718 w4719 _ w4720 w4721 w4722 w4723 w4724 w4725 _]
                frame 0 {
                  n3384 = local write "S"(w4570) -> ()
                }
                frame 1 {
                  n3385 = local write "S 2"(w4571) -> ()
                }
                frame 2 {
                }
                frame 3 {
                  n3386 = local write "S 4"(w4572) -> ()
                }
                frame 4 {
                  n3387 = property on="FILE" class="Str"("Caption.Text"=w4573) -> ()  [unwired: 2 in, 2 out]
                }
                frame 5 {
                  n3388 = property on="Fuel Discription :" class="Str"("Caption.Text"=w4574) -> ()  [unwired: 2 in, 2 out]
                }
                frame 6 {
                  n3389 = property on="Remarks :" class="Str"("Caption.Text"=w4575) -> ()  [unwired: 2 in, 2 out]
                }
                frame 7 {
                  n3390 = property on="Save & Continue" class="Bool (strict)"("Boolean Text.Text"=w4576) -> ()  [unwired: 2 in, 2 out]
                }
                frame 8 {
                }
                frame 9 {
                  n3391 = property on="Set Hz" class="DigNum (strict)"("Caption.Text"=w4578) -> ()  [unwired: 2 in, 2 out]
                }
                frame 10 {
                  "String 3" <- w4579
                }
                frame 11 {
                  n3392 = property on="NORMAL LOAD" class="DigNum (strict)"("Caption.Text"=w4580) -> ()  [unwired: 2 in, 2 out]
                }
                frame 12 {
                  "String 5" <- w4581
                }
                frame 13 {
                  n3393 = property on="Set Temp" class="DigNum (strict)"("Caption.Text"=w4582) -> ()  [unwired: 2 in, 2 out]
                }
                frame 14 {
                  n3394 = local write "S 15"(w4583) -> ()
                }
                frame 15 {
                  n3395 = property on="Set Rh" class="DigNum (strict)"("Caption.Text"=w4584) -> ()  [unwired: 2 in, 2 out]
                }
                frame 16 {
                  "String 13" <- w4585
                  "String 26" <- w4585
                }
                frame 17 {
                  n3396 = local write "S 18"(w4586) -> ()
                }
                frame 18 {
                  "String 17" <- w4587
                }
                frame 19 {
                  n3397 = property on="test time" class="DigNum (strict)"("Caption.Text"=w4588) -> ()  [unwired: 2 in, 2 out]
                }
                frame 20 {
                  "String 18" <- w4589
                  "String 22" <- w4589
                }
                frame 21 {
                  n3398 = property on="Elapsed time" class="DigNum (strict)"("Caption.Text"=w4590) -> ()  [unwired: 2 in, 2 out]
                }
                frame 22 {
                  n3399 = property on="Samplingtime 2" class="DigNum (strict)"("Caption.Text"=w4591) -> ()  [unwired: 2 in, 2 out]
                }
                frame 23 {
                  "String 21" <- w4592
                }
                frame 24 {
                  n3400 = property on="Countdown" class="DigNum (strict)"("Caption.Text"=w4593) -> ()  [unwired: 2 in, 2 out]
                }
                frame 25 {
                  n3401 = property on="Countdown 2" class="DigNum (strict)"("Caption.Text"=w4594) -> ()  [unwired: 2 in, 2 out]
                }
                frame 26 {
                  n3402 = property on="Engage" class="Bool (strict)"("Boolean Text.Text"=w4595) -> ()  [unwired: 2 in, 2 out]
                }
                frame 27 {
                  n3403 = property on="Boolean  4" class="Bool (strict)"("Boolean Text.Text"=w4596) -> ()  [unwired: 2 in, 2 out]
                }
                frame 28 {
                  n3404 = property on="Test \nStatus" class="Bool (strict)"("Boolean Text.Text"=w4597) -> ()  [unwired: 2 in, 2 out]
                }
                frame 29 {
                }
                frame 30 {
                }
                frame 31 {
                }
                frame 32 {
                  n3405 = property on="RSTCOF" class="Bool"("Boolean Text.Text"=w4599) -> ()  [unwired: 2 in, 2 out]
                  n3406 = property on="RST FF" class="Bool"("Boolean Text.Text"=w4599) -> ()  [unwired: 2 in, 2 out]
                  n3407 = property on="RST TEMP" class="Bool"("Boolean Text.Text"=w4599) -> ()  [unwired: 2 in, 2 out]
                  n3408 = property on="RSTV1 3" class="Bool"("Boolean Text.Text"=w4599) -> ()  [unwired: 2 in, 2 out]
                  n3409 = property on="rstv2" class="Bool"("Boolean Text.Text"=w4599) -> ()  [unwired: 2 in, 2 out]
                  n3410 = property on="RSTV1 2" class="Bool"("Boolean Text.Text"=w4599) -> ()  [unwired: 2 in, 2 out]
                  n3411 = property on="RST CP" class="Bool"("Boolean Text.Text"=w4599) -> ()  [unwired: 2 in, 2 out]
                }
                frame 33 {
                  "S 61" <- w4600
                }
                frame 34 {
                  "String 23" <- w4601
                }
                frame 35 {
                  n3412 = property on="Rh Before" class="DigNum (strict)"("Caption.Text"=w4602) -> ()  [unwired: 2 in, 2 out]
                }
                frame 36 {
                  n3413 = Match Pattern(string=w4603, regular expression=",") -> (before substring=→"bs":string, after substring=→"as":string)  [unwired: 1 in, 2 out]
                  n3414 = property on="Rh After" class="DigNum (strict)"("Caption.Text"=w4603) -> ()  [unwired: 2 in, 2 out]
                }
                frame 37 {
                  n3415 = Match Pattern(string=w4612, regular expression=",") -> (before substring=w4611:string, after substring=w4610:string)  [unwired: 1 in, 2 out]
                  "bs" <- w4611
                  "as" <- w4610
                  n3416 = Concatenate Strings(w4611, w4610) -> (w4607:string)
                  n3417 = property on="Humidity before test 2" class="DigNum (strict)"("Caption.Text"=w4607) -> ()  [unwired: 2 in, 2 out]
                  n3418 = property on="Humidity before test" class="DigNum (strict)"("Caption.Text"=w4607) -> ()  [unwired: 2 in, 2 out]
                  n3419 = Concatenate Strings(w4607, "=" ("string")) -> (w4608:string)
                  n3420 = local write "S 38"(w4608) -> ()
                }
                frame 38 {
                  n3421 = Match Pattern(string=w4619, regular expression=",") -> (before substring=w4618:string, after substring=w4617:string)  [unwired: 1 in, 2 out]
                  "bs" <- w4618
                  "as" <- w4617
                  n3422 = Concatenate Strings(w4618, w4617) -> (w4614:string)
                  n3423 = property on="Humidity after test 2" class="DigNum (strict)"("Caption.Text"=w4614) -> ()  [unwired: 2 in, 2 out]
                  n3424 = Concatenate Strings(w4614, "=" ("string")) -> (w4616:string)
                  n3425 = property on="Humidity after test" class="DigNum (strict)"("Caption.Text"=w4614) -> ()  [unwired: 2 in, 2 out]
                  n3426 = local write "S 39"(w4616) -> ()
                }
                frame 39 {
                  n3427 = Match Pattern(string=w4626, regular expression=",") -> (before substring=w4625:string, after substring=w4624:string)  [unwired: 1 in, 2 out]
                  "bs" <- w4625
                  "as" <- w4624
                  n3428 = Concatenate Strings(w4625, w4624) -> (w4621:string)
                  n3429 = property on="Temperature before test 2" class="DigNum (strict)"("Caption.Text"=w4621) -> ()  [unwired: 2 in, 2 out]
                  n3430 = property on="Temperature before test" class="DigNum (strict)"("Caption.Text"=w4621) -> ()  [unwired: 2 in, 2 out]
                  n3431 = Concatenate Strings(w4621, "=" ("string")) -> (→"String 34":string)
                }
                frame 40 {
                  n3432 = Match Pattern(string=w4633, regular expression=",") -> (before substring=w4632:string, after substring=w4631:string)  [unwired: 1 in, 2 out]
                  "bs" <- w4632
                  "as" <- w4631
                  n3433 = Concatenate Strings(w4632, w4631) -> (w4628:string)
                  n3434 = property on="Temperature after test 2" class="DigNum (strict)"("Caption.Text"=w4628) -> ()  [unwired: 2 in, 2 out]
                  n3435 = Concatenate Strings(w4628, "=" ("string")) -> (→"String 35":string)
                  n3436 = property on="Temperature after test" class="DigNum (strict)"("Caption.Text"=w4628) -> ()  [unwired: 2 in, 2 out]
                }
                frame 41 {
                  n3437 = property on="AVP" class="DigNum (strict)"("Caption.Text"=w4637) -> ()  [unwired: 2 in, 2 out]
                  n3438 = property on="AVP 2" class="DigNum (strict)"("Caption.Text"=w4637) -> ()  [unwired: 2 in, 2 out]
                  n3439 = Concatenate Strings(w4637, "=" ("string")) -> (→"String 36":string)
                }
                frame 42 {
                  n3440 = property on="MWSD" class="DigNum (strict)"("Caption.Text"=w4640) -> ()  [unwired: 2 in, 2 out]
                  n3441 = property on="MWSD 2" class="DigNum (strict)"("Caption.Text"=w4640) -> ()  [unwired: 2 in, 2 out]
                  n3442 = Concatenate Strings(w4640, "=" ("string")) -> (→"String 37":string)
                }
                frame 43 {
                  n3443 = property on="HCF 2" class="DigNum (strict)"("Caption.Text"=w4643) -> ()  [unwired: 2 in, 2 out]
                  n3444 = property on="HCF" class="DigNum (strict)"("Caption.Text"=w4643) -> ()  [unwired: 2 in, 2 out]
                  n3445 = Concatenate Strings(w4643, "=" ("string")) -> (→"String 38":string)
                }
                frame 44 {
                  n3446 = Concatenate Strings(w4645, "=" ("string")) -> (→"String 39":string)
                  n3447 = property on="WS1.4 2" class="DigNum (strict)"("Caption.Text"=w4645) -> ()  [unwired: 2 in, 2 out]
                  n3448 = property on="WS1.4" class="DigNum (strict)"("Caption.Text"=w4645) -> ()  [unwired: 2 in, 2 out]
                }
                frame 45 {
                  n3449 = property on="Save Results" class="Bool (strict)"("Boolean Text.Text"=w4647) -> ()  [unwired: 2 in, 2 out]
                }
                frame 46 {
                  n3450 = local write "S 47"(w4648) -> ()
                }
                frame 47 {
                  n3451 = local write "S 48"(w4649) -> ()
                }
                frame 48 {
                  n3452 = local write "S 49"(w4650) -> ()
                }
                frame 49 {
                  n3453 = local write "S 50"(w4651) -> ()
                }
                frame 50 {
                  n3454 = local write "S 51"(w4652) -> ()
                }
                frame 51 {
                  n3455 = local write "S 52"(w4653) -> ()
                }
                frame 52 {
                  n3456 = local write "S 53"(w4654) -> ()
                }
                frame 53 {
                  n3457 = local write "S 54"(w4655) -> ()
                }
                frame 54 {
                  n3458 = local write "S 55"(w4656) -> ()
                }
                frame 55 {
                  n3459 = local write "S 56"(w4657) -> ()
                }
                frame 56 {
                  n3460 = local write "S 57"(w4658) -> ()
                }
                frame 57 {
                  n3461 = local write "S 58"(w4659) -> ()
                }
                frame 58 {
                  n3462 = local write "S 59"(w4660) -> ()
                }
                frame 59 {
                  n3463 = local write "S 60"(w4661) -> ()
                }
                frame 60 {
                  n3464 = local write "S 62"(w4662) -> ()
                }
                frame 61 {
                  n3465 = local write "S 63"(w4663) -> ()
                }
                frame 62 {
                  n3466 = local write "S 64"(w4664) -> ()
                }
                frame 63 {
                  n3467 = local write "S 65"(w4665) -> ()
                }
                frame 64 {
                  n3468 = local write "S 66"(w4666) -> ()
                }
                frame 65 {
                  n3469 = local write "S 67"(w4667) -> ()
                }
                frame 66 {
                  n3470 = local write "S 68"(w4668) -> ()
                }
                frame 67 {
                  n3471 = local write "S 69"(w4669) -> ()
                }
                frame 68 {
                  n3472 = local write "S 70"(w4670) -> ()
                }
                frame 69 {
                  n3473 = local write "S 71"(w4671) -> ()
                }
                frame 70 {
                  n3474 = local write "S 72"(w4672) -> ()
                }
                frame 71 {
                  n3475 = local write "S 73"(w4673) -> ()
                }
                frame 72 {
                  n3476 = local write "S 74"(w4674) -> ()
                }
                frame 73 {
                  n3477 = local write "S 75"(w4675) -> ()
                }
                frame 74 {
                  n3478 = local write "S 76"(w4676) -> ()
                }
                frame 75 {
                  n3479 = local write "S 77"(w4677) -> ()
                }
                frame 76 {
                  n3480 = local write "S 78"(w4678) -> ()
                }
                frame 77 {
                  n3481 = local write "S 79"(w4679) -> ()
                }
                frame 79 {
                  n3482 = property on="Sample Temperature ( °C )" class="XYGraph (strict)"("Y Scale.Name Label.Text"=w4680) -> ()  [unwired: 2 in, 2 out]
                }
                frame 80 {
                  n3483 = local write "S 81"(w4681) -> ()
                  n3484 = property on="Humidity ( %RH )" class="XYGraph (strict)"("Y Scale.Name Label.Text"=w4681) -> ()  [unwired: 2 in, 2 out]
                }
                frame 78 {
                  n3485 = property on="Air Temperature  ( °C )" class="XYGraph (strict)"("X Scale.Name Label.Text"=w4682) -> ()  [unwired: 2 in, 2 out]
                  n3486 = property on="Humidity ( %RH )" class="XYGraph (strict)"("X Scale.Name Label.Text"=w4682) -> ()  [unwired: 2 in, 2 out]
                  n3487 = property on="Sample Temperature ( °C )" class="XYGraph (strict)"("X Scale.Name Label.Text"=w4682) -> ()  [unwired: 2 in, 2 out]
                  n3488 = property on="Coefficient Of Friction" class="XYGraph (strict)"("X Scale.Name Label.Text"=w4682) -> ()  [unwired: 2 in, 2 out]
                }
                frame 81 {
